vi "Stop Stream.vi"(8 "error in (no error)":errorcluster, 10 "stream index":i32, 11 "refnum in":refnum<k20>) -> (0 "error out":errorcluster, 1 "samples transferred":u64, 2 "stream state":T1, 3 "refnum out":refnum<k20>)   [LabVIEW 2015, in "niInstr Streaming v1 Host.lvlib"]
doc: "Stops the specified stream by commanding it into a Cancelled state. Stopping a stream does not necessarily flush samples that may be in flight in a FIFO. Care should be taken to ensure that abandoned samples are discarded. Calling Stop and Start on a FIFO primitive is one such way to abandon in-flight samples. A user may also read all remaining samples from a Target to Host FIFO.\n\nUpon Cancelling the stream, the num samples transferred value stops incrementing and accurately represents the final state of the transfer. If the stream is in a healthy state when the cancellation request is issued, it shall enter the cancelled state. If the stream is in an error state (Error), the stream shall not exit the Error state in response to the cancellation so that errors can be properly noted.\n\nError states can only be left by using the Clear Stream.vi\n\n<B>Input Parameters</B>\n\n<B>error in (no error)</B> 'error in' can accept error information wired from VIs previously called. Use this information to decide if any functionality should be bypassed in the event of errors from other VIs.\n\nRight-click the 'error in' control on the front panel and select 'Explain Error' or 'Explain Warning' from the shortcut menu for more information about the error.\n\n<B>stream index</B> Selects which stream index this VI will interface to. This is the index number at the end of the host interface controls (0..7).\n\n<B>refnum in</B> Wire in the session obtained from Open FPGA Reference.\n\n<B>Output Parameters</B>\n\n<B>error out</B> contains error information. This output provides standard error out functionality.\n\n<B>refnum out</B> Copy of refnum in"
uses:
  <instrlib>/_niInstr/Streaming/v1/Host/niInstr Streaming v1 Host.lvlib
  <instrlib>/_niInstr/Streaming/v1/Common/Stream State.ctl
  <instrlib>/_niInstr/Streaming/v1/Common/niInstr Streaming v1 Common.lvlib
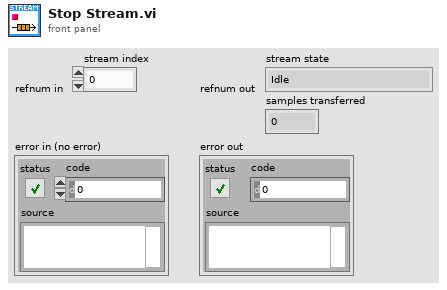
[diagram p1: front panel]
types:
  T1 = typedef "niInstr Streaming v1 Common.lvlib/Stream State.ctl" = enum8{"Idle", "Finite Transfer", "Continuous", "Done", "Error", "Not Ready", "Cancel"}
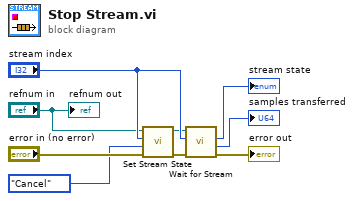
[diagram p0: block diagram]
diagram:
  n1 = call <instrlib>:"Set Stream State.vi"("error in (no error)"="error in (no error)", "stream state"=Stream_State."Cancel" ("stream.request state 0"), "stream index"="stream index", "refnum in"="refnum in") -> ("error out"=w6:errorcluster, "refnum out"=w1:refnum<k20>)  [unwired: 6 in]
  n2 = call <instrlib>:"Wait for Stream.vi"("error in (no error)"=w6, "stream index"="stream index", "refnum in"=w1) -> ("error out"=→"error out":errorcluster, "samples transferred"=→"samples transferred":u64, "stream state"=→"stream state":T1)  [unwired: 5 in, 1 out]
  "refnum out" <- "refnum in"
